vi "validate.vi"(8 "error in":errorcluster, 11 "EthernetIP configuration in":refnum<class "EIP Tags Configuration.lvclass">) -> (0 "error out":errorcluster, 3 "EthernetIP configuration out":refnum<class "EIP Tags Configuration.lvclass">)   [LabVIEW 2013, in "EIP Tags Configuration.lvclass"]
doc: "This function performs validation of the configuration. This function should be safe to call at any point and should not rely on anything in the runtime environment."
uses:
  EIP Tags Configuration.lvclass
  <vilib>/NI/Tag Bus Module Framework/module configuration/TBM module configuration.lvclass
  EIP Tags Configuration.lvclass/EIP Tags Configuration.ctl
  channel/EIP Tags Channel.lvclass/EIP Tags Channel.ctl
  channel/Read element.vi
  channel/Read EIP Tag UUID.vi
  channel/EIP Tags Channel.lvclass
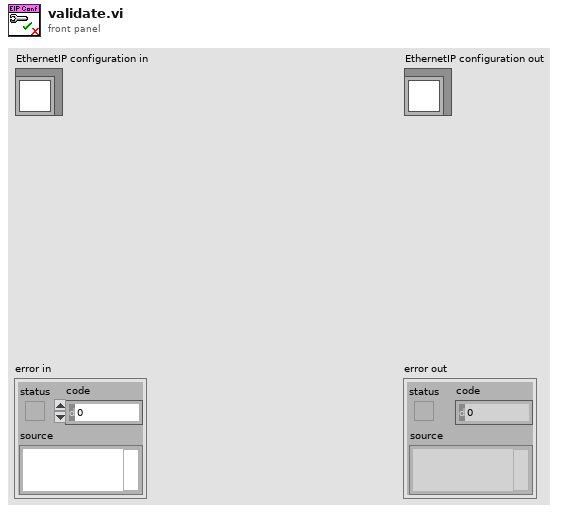
[diagram p1: front panel]
types:
  T1 = typedef "EIP Tags Configuration.lvclass/eip tag definition.ctl" = cluster{"eip tag types":T2, "unique tag name":string, "Number of Elements":u32}
  T2 = typedef "EIP Tags Configuration.lvclass/eip tag types.ctl" = enum16{"SINT", "INT", "DINT", "REAL", "BOOL", "STRING"}
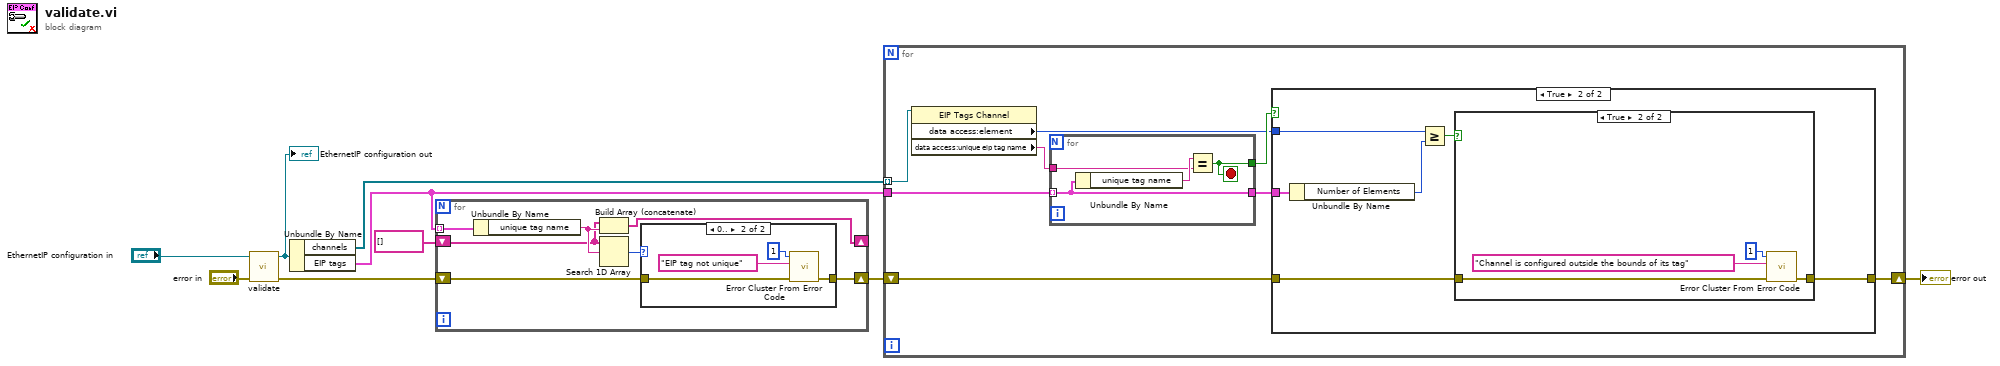
[diagram p0: block diagram]
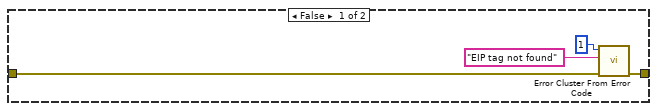
[diagram p2: hidden frame]
diagram:
  n1 = call-parent "validate.vi"("error in"="error in", "configuration in"="EthernetIP configuration in") -> ("error out"=w5:errorcluster, "configuration out"=w7:refnum<class "EIP Tags Configuration.lvclass">)  [unwired: 8 in]
  "EthernetIP configuration out" <- w7
  n2 = Unbundle By Name(w7) -> ("channels"=w4:refnum<class "EIP Tags Channel.lvclass">[], "EIP tags"=w3:T1[])
  n3 = for {
    tunnel: w3 -> [w16] mode=indexing
    shift-right: [w15] -> _
    shift-left: string[] [] -> [w13]
    shift-right: [w11] -> w2
    shift-left: w5 -> [w12]
    n4 = Unbundle By Name(w16) -> ("unique tag name"=w14:string)
    n5 = Build Array (concatenate)(w13, w14) -> (w15:string[])
    n6 = Search 1D Array(1D array=w13, element=w14) -> (index of element=w10:i32)  [unwired: 1 in]
    n7 = case shown="0.." w10 {
      tunnel: w12 -> [w17 w20]
      tunnel: [w17 w21] -> w11
      frame ..-1 {
      }
      frame 0.. {
        n8 = call <vilib>:"Error Cluster From Error Code.vi"("error in (no error)"=w20, "error message (\"\")"="EIP tag not unique" ("error message (\"\")"), "error code (0)"=1) -> ("error out"=w21:errorcluster)  [unwired: 6 in]
      }
    }
  }
  n9 = for {
    tunnel: w4 -> [w28] mode=indexing
    tunnel: w3 -> [w29]
    shift-right: [w23] -> w1
    shift-left: w2 -> [w24]
    n10 = property class="EIP Tags Channel"(reference=w28) -> ("data access:element"=w22:i32, "data access:unique eip tag name"=w27:string)  [unwired: 1 in, 2 out]
    n11 = for {
      tunnel: w29 -> [w46] mode=indexing
      tunnel: w27 -> [w47]
      tunnel: [w46] -> w25
      tunnel: [w45] -> w26
      stop <- w45 stop-if-true
      n12 = Unbundle By Name(w46) -> ("unique tag name"=w48:string)
      n13 = Equal?(x=w48, y=w47) -> (x = y?=w45:bool)
    }
    n14 = case shown="True" w26 {
      tunnel: w25 -> [_ w39]
      tunnel: w24 -> [w32 w35]
      tunnel: [w31 w36] -> w23
      tunnel: w22 -> [_ w34]
      frame False {
        n15 = call <vilib>:"Error Cluster From Error Code.vi"("error in (no error)"=w32, "error message (\"\")"="EIP tag not found" ("error message (\"\")"), "error code (0)"=1) -> ("error out"=w31:errorcluster)  [unwired: 6 in]
      }
      frame True {
        n16 = Unbundle By Name(w39) -> ("Number of Elements"=w38:u32)
        n17 = Greater Or Equal?(x=w34, y=w38) -> (x >= y?=w37:bool)
        n18 = case shown="True" w37 {
          tunnel: [w40 w41] -> w36
          tunnel: w35 -> [w40 w42]
          frame False {
          }
          frame True {
            n19 = call <vilib>:"Error Cluster From Error Code.vi"("error in (no error)"=w42, "error message (\"\")"="Channel is configured outside the bounds of its tag" ("error message (\"\")"), "error code (0)"=1) -> ("error out"=w41:errorcluster)  [unwired: 6 in]
          }
        }
      }
    }
  }
  "error out" <- w1
